vi "Run Sequence.vi"(0 "XNET Sesion":refnum<k21>, 2 "Barcode":string, 11 "Error In":errorcluster) -> (4 "Pass":bool, 15 "Error Out":errorcluster)   [LabVIEW 2021]
doc: "Runs the actual IPC flash sequence. It will only pass if the DUT reports PCBAID 5 and Geneology reads back successfully."
uses:
  Controls/Sequence States.ctl
  Controls/Console Manager Functions.ctl
  Lunar Libraries/UDS CAN/Controls/UDSSessionParameters.ctl
  <vilib>/xnet/xnet.llb/XNET Create Session (Signal Input Single-point).vi
  Global Variable.vi
  <vilib>/regexp/Match Regular Expression.xnode
  <vilib>/xnet/xnet.llb/XNET Read (Signal Single-point).vi
  Lunar Libraries/UDS CAN/Lunar UDS CAN.lvlib
  Lunar Libraries/PCAN Reader/PCAN Reader.lvlib
panel:
  # "Inputs"
  # "Outputs"
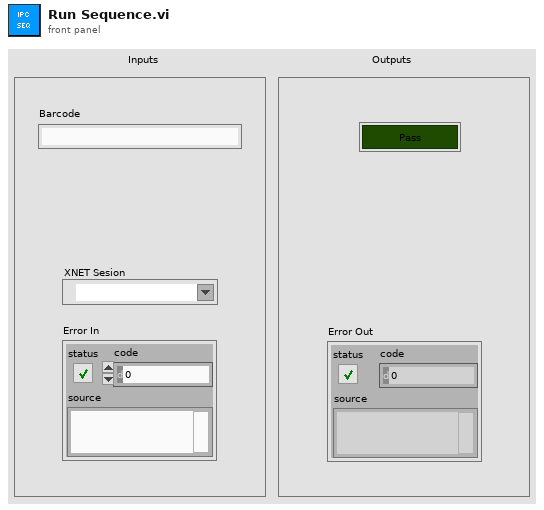
[diagram p1: front panel]
types:
  T1 = typedef "Sequence States.ctl" = enum16{"Check Barcode", "Check PCBAID", "Flash BL", "Confirm PCBAID", "Genealogy"}
  T2 = typedef "Console Manager Functions.ctl" = enum16{"Init", "Add", "Get"}
  T3 = typedef "Lunar UDS CAN.lvlib/UDSSessionParameters.ctl" = cluster{"XNET Interface":string, "BaudRate":u64, "Transmit ID":i32, "Receive ID":i32}
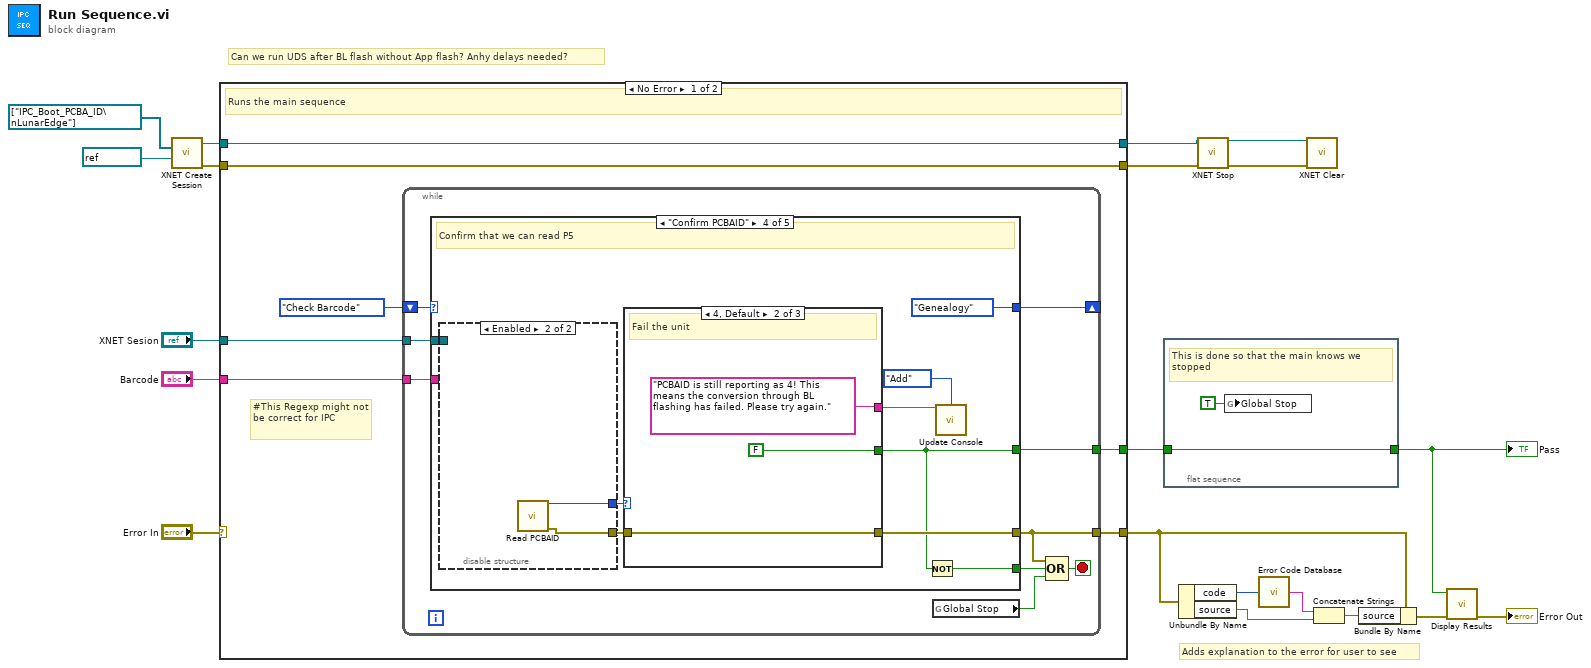
[diagram p0: block diagram]
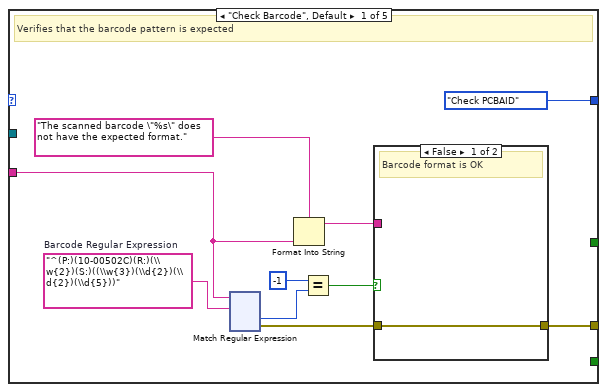
[diagram p2: hidden frame]
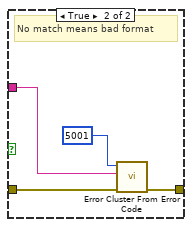
[diagram p3: hidden frame]
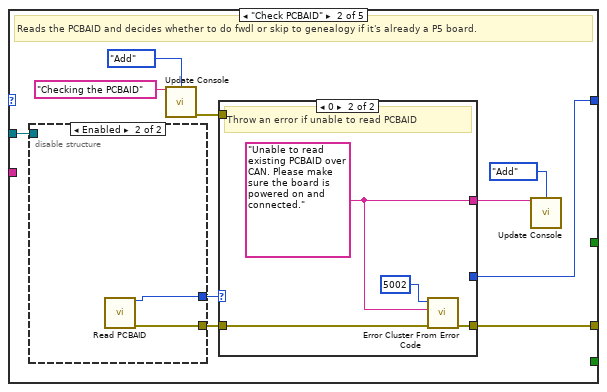
[diagram p4: hidden frame]
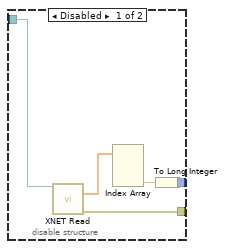
[diagram p5: hidden frame]
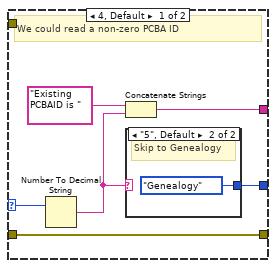
[diagram p6: hidden frame]
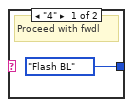
[diagram p7: hidden frame]
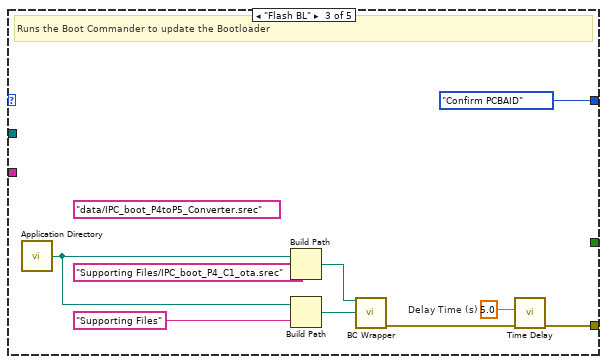
[diagram p8: hidden frame]
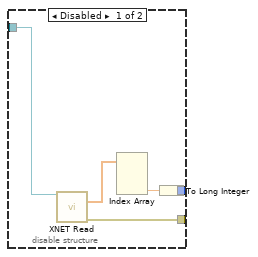
[diagram p9: hidden frame]
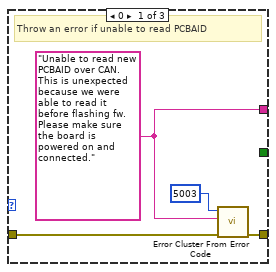
[diagram p10: hidden frame]
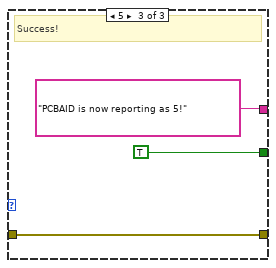
[diagram p11: hidden frame]
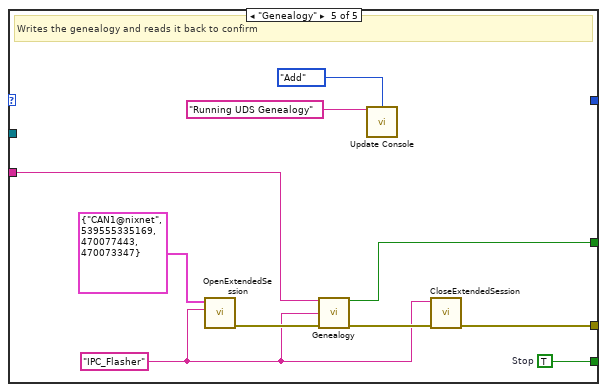
[diagram p12: hidden frame]
diagram:
  # "Can we run UDS after BL flash without App flash? Anhy delays needed?"
  # "Adds explanation to the error for user to see"
  n1 = call-poly <vilib>:"XNET Create Session.vi"("signal list"=refnum<k21>[] ["IPC_Boot_PCBA_ID\nLunarEdge"], "interface"=refnum<k21> "CAN1") -> ("session out"=w6:refnum<k21>, "error out"=w7:errorcluster)  [unwired: 12 in]
  n2 = case shown="No Error" "Error In" {
    selector: "Error In" -> [_ w245]
    tunnel: "Barcode" -> [w27 _]
    tunnel: [w26 w245] -> w14
    tunnel: "XNET Sesion" -> [w24 _]
    tunnel: [w23 _] -> w1
    tunnel: [w22 w243] -> w8
    tunnel: w7 -> [w22 w243]
    tunnel: w6 -> [w21 w244]
    tunnel: [w21 w244] -> w5
    frame No Error {
      # "#This Regexp might not be correct for IPC"
      # "Runs the main sequence"
      n3 = while {
        shift-right: [w34] -> _
        shift-left: Sequence_States."Check Barcode" -> [w36]
        tunnel: w27 -> [w35]
        tunnel: [w31] -> w26
        tunnel: w24 -> [w33]
        tunnel: [w32] -> w23
        stop <- w30 stop-if-true
        n4 = case shown="\"Confirm PCBAID\"" w36 {
          tunnel: w35 -> [w37 _ _ _ w237]
          tunnel: [w41 w175 w204 w212 w241] -> w31
          tunnel: [Sequence_States."Check PCBAID" w174 Sequence_States."Confirm PCBAID" Sequence_States."Genealogy" _] -> w34
          tunnel: w33 -> [_ w178 _ w215 _]
          tunnel: [_ _ _ w208 w236] -> w32
          tunnel: [_ _ _ w207 w242] -> w29
          frame "Check Barcode", Default {
            w46 = "^(P:)(10-00502C)(R:)(\\w{2})(S:)((\\w{3})(\\d{2})(\\d{2})(\\d{5}))"  # Barcode Regular Expression
            # "Verifies that the barcode pattern is expected"
            n5 = xnode "Match Regular Expression"("input string"=w37, "regular expression"=w46) -> ("offset past match"=w45:i32, "error out"=w42:errorcluster)  [unwired: 4 in, 3 out]
            n6 = Format Into String(format string="The scanned barcode \"%s\" does not have the expected format.", w37) -> (resulting string=w38:string)  [unwired: 2 in, 1 out]
            n7 = Equal?(x=-1, y=w45) -> (x = y?=w40:bool)
            n8 = case shown="False" w40 {
              tunnel: w42 -> [w47 w51]
              tunnel: [w47 w50] -> w41
              tunnel: w38 -> [_ w48]
              frame False {
                # "Barcode format is OK"
              }
              frame True {
                # "No match means bad format"
                n9 = call <vilib>:"Error Cluster From Error Code.vi"("error in (no error)"=w51, "error message (\"\")"=w48, "error code (0)"=5001) -> ("error out"=w50:errorcluster)  [unwired: 6 in]
              }
            }
          }
          frame "Check PCBAID" {
            # "Reads the PCBAID and decides whether to do fwdl or skip to genealogy if it's already a P5 board."
            n10 = disable-structure shown="Enabled" {
              disable-tunnel: w178 -> [w183 _]
              disable-tunnel: [w180 w184] -> w177
              disable-tunnel: [w179 w185] -> w176
              frame Disabled {
                n11 = call-poly <vilib>:"XNET Read.vi"("session in"=w183) -> ("data"=w182:dbl[], "error out"=w179:errorcluster)  [unwired: 12 in, 1 out]
                n12 = Index Array(array=w182) -> (element #3=w181:dbl)  [unwired: 3 in, 2 out]
                n13 = To Long Integer(number=w181) -> (32bit integer=w180:i32)
              }
              frame Enabled {
                n14 = call "Read PCBAID.vi"() -> ("PCBAID"=w184:u8, "Error Out"=w185:errorcluster)  [unwired: 14 in]
              }
            }
            n15 = call "Update Console.vi"("New Line"="Checking the PCBAID", "Function"=Console_Manager_Functions."Add") -> ("Error Out"=w169:errorcluster)  [unwired: 12 in, 1 out]
            n16 = case shown="0" w177 {
              selector: w177 -> [w190 _]
              tunnel: w176 -> [w189 w197]
              tunnel: [w189 w196] -> w175
              tunnel: [w187 _] -> w174
              tunnel: [w186 w194] -> w173
              tunnel: w169 -> [_ _]
              frame 4, Default {
                # "We could read a non-zero PCBA ID"
                n17 = Number To Decimal String(number=w190) -> (decimal integer string=w188:string)  [unwired: 1 in]
                n18 = Concatenate Strings("Existing PCBAID is ", w188) -> (w186:string)
                n19 = case shown="\"5\", Default" w188 {
                  tunnel: [Sequence_States."Flash BL" Sequence_States."Genealogy"] -> w187
                  frame "4" {
                    # "Proceed with fwdl"
                  }
                  frame "5", Default {
                    # "Skip to Genealogy"
                  }
                }
              }
              frame 0 {
                w194 = "Unable to read existing PCBAID over CAN. Please make sure the board is powered on and connected."
                # "Throw an error if unable to read PCBAID"
                n20 = call <vilib>:"Error Cluster From Error Code.vi"("error in (no error)"=w197, "error message (\"\")"=w194, "error code (0)"=5002) -> ("error out"=w196:errorcluster)  [unwired: 6 in]
              }
            }
            n21 = call "Update Console.vi"("New Line"=w173, "Function"=Console_Manager_Functions."Add") -> ()  [unwired: 12 in, 2 out]
          }
          frame "Flash BL" {
            (unwired) "data/IPC_boot_P4toP5_Converter.srec"
            w203 = 5.0  # Delay Time (s)
            # "Runs the Boot Commander to update the Bootloader"
            n22 = call <vilib>:"Application Directory.vi"() -> ("Application Directory"=w200:path)
            n23 = Build Path(base path=w200, name or relative path="Supporting Files/IPC_boot_P4_C1_ota.srec") -> (appended path=w201:path)
            n24 = Build Path(base path=w200, name or relative path="Supporting Files") -> (appended path=w202:path)
            n25 = call "BC Wrapper.vi"("File To Program"=w201, "BootCommander Folder"=w202) -> ("error out"=w205:errorcluster)  [unwired: 11 in, 2 out]
            n26 = call "Time Delay"("error in (no error)"=w205, "Delay Time (s)"=w203) -> ("error out"=w204:errorcluster)  [unwired: 9 in]
          }
          frame "Confirm PCBAID" {
            # "Confirm that we can read P5"
            n27 = disable-structure shown="Enabled" {
              disable-tunnel: w215 -> [w220 _]
              disable-tunnel: [w217 w222] -> w214
              disable-tunnel: [w216 w221] -> w213
              frame Disabled {
                n28 = call-poly <vilib>:"XNET Read.vi"("session in"=w220) -> ("data"=w219:dbl[], "error out"=w216:errorcluster)  [unwired: 12 in, 1 out]
                n29 = Index Array(array=w219) -> (element #3=w218:dbl)  [unwired: 3 in, 2 out]
                n30 = To Long Integer(number=w218) -> (32bit integer=w217:i32)
              }
              frame Enabled {
                n31 = call "Read PCBAID.vi"() -> ("PCBAID"=w222:u8, "Error Out"=w221:errorcluster)  [unwired: 14 in]
              }
            }
            n32 = case shown="4, Default" w214 {
              tunnel: [w223 "PCBAID is still reporting as 4! This means the conversion through BL flashing has failed. Please try again." "PCBAID is now reporting as 5!"] -> w210
              tunnel: w213 -> [w226 w228 w231]
              tunnel: [w225 w228 w231] -> w212
              tunnel: [_ FALSE TRUE] -> w208
              frame 0 {
                w223 = "Unable to read new PCBAID over CAN. This is unexpected because we were able to read it before flashing fw. Please make sure the board is powered on and connected."
                # "Throw an error if unable to read PCBAID"
                n33 = call <vilib>:"Error Cluster From Error Code.vi"("error in (no error)"=w226, "error message (\"\")"=w223, "error code (0)"=5003) -> ("error out"=w225:errorcluster)  [unwired: 6 in]
              }
              frame 4, Default {
                # "Fail the unit"
              }
              frame 5 {
                # "Success!"
              }
            }
            n34 = Not(x=w208) -> (.not. x?=w207:bool)
            n35 = call "Update Console.vi"("New Line"=w210, "Function"=Console_Manager_Functions."Add") -> ()  [unwired: 12 in, 2 out]
          }
          frame "Genealogy" {
            w235 = "IPC_Flasher" ("SessionID")
            w242 = TRUE  # Stop
            # "Writes the genealogy and reads it back to confirm"
            n36 = call "OpenExtendedSession.vi"("SessionID"=w235, "UDS Session Parameters"=T3 {"XNET Interface"="CAN1@nixnet", "BaudRate"=539555335169, "Transmit ID"=470077443, "Receive ID"=470073347}) -> ("error out"=w239:errorcluster)  [unwired: 9 in]
            n37 = call "Genealogy.vi"("Barcode"=w237, "SessionID"=w235, "Error In"=w239) -> ("Pass"=w236:bool, "Error Out"=w238:errorcluster)  [unwired: 11 in]
            n38 = call "Update Console.vi"("New Line"="Running UDS Genealogy" ("Value (Signaling)"), "Function"=Console_Manager_Functions."Add") -> ()  [unwired: 12 in, 2 out]
            n39 = call "CloseExtendedSession.vi"("error in (no error)"=w238, "SessionID"=w235) -> ("error out"=w241:errorcluster)  [unwired: 9 in]
          }
        }
        n40 = global read "Global Variable.vi" "Global Stop"() -> (w28:bool)
        n41 = Compound Arithmetic op=OR(w31, w29, w28) -> (w30:bool)
      }
    }
    frame Error {
      # "Can't start due to error"
    }
  }
  n42 = flat-sequence {
    tunnel: [w247] -> w2
    tunnel: w1 -> [w247]
    frame #0 {
      # "This is done so that the main knows we stopped"
      n43 = global write "Global Variable.vi" "Global Stop"(TRUE ("Global Stop")) -> ()
    }
  }
  n44 = Unbundle By Name(w14) -> ("code"=w18:i32, "source"=w17:string)
  n45 = call <vilib>:"XNET Stop.vi"("session in"=w5, "error in (no error)"=w8) -> ("session out"=w9:refnum<k21>, "error out"=w10:errorcluster)  [unwired: 12 in]
  n46 = call <vilib>:"Error Code Database.vi"("Error Code"=w18) -> ("Error Text"=w16:string)
  n47 = call <vilib>:"XNET Clear.vi"("session in"=w9, "error in (no error)"=w10) -> ()  [unwired: 13 in, 1 out]
  n48 = Concatenate Strings(w16, w17) -> (w15:string)
  n49 = Bundle By Name(cluster=w14, "source"=w15) -> (w4:errorcluster)
  n50 = call "Display Results.vi"("Error In"=w4, "Pass"=w2) -> ("Error Out"=→"Error Out":errorcluster)  [unwired: 9 in]
  "Pass" <- w2
